vi "DisposeCore.vi"(8 "error in (no error)":errorcluster, 11 "ChicagoStylePepperoniPizza":refnum<class "ChicagoStylePepperoniPizza.lvclass">) -> (0 "error out":errorcluster, 3 "ChicagoStylePepperoniPizza":refnum<class "ChicagoStylePepperoniPizza.lvclass">)   [LabVIEW 2020, in "FactoryMethod.lvlib" / "PizzaFactoryMethod.lvlib" / "ChicagoStylePepperoniPizza.lvclass"]
uses:
  ChicagoStylePepperoniPizza.lvclass
  ChicagoStylePepperoniPizza.lvclass/ChicagoStylePepperoniPizza.ctl
  Private/TypeDef/privateDataDVR.ctl
  Private/TypeDef/privateData.ctl
  Pizza/Pizza.lvclass
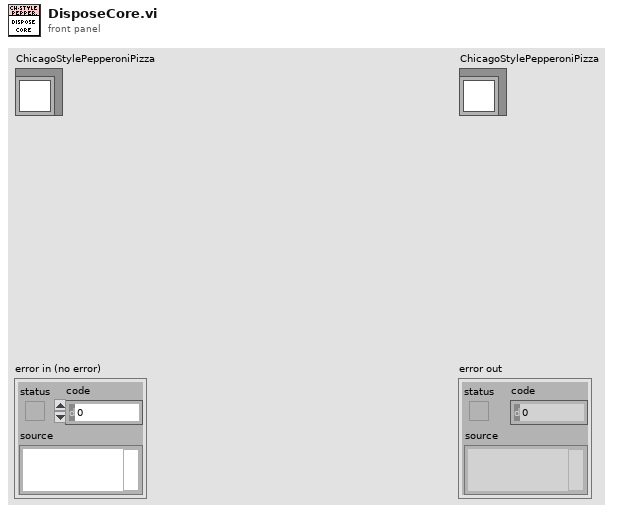
[diagram p1: front panel]
types:
  T1 = typedef "FactoryMethod.lvlib/PizzaFactoryMethod.lvlib/ChicagoStylePepperoniPizza.lvclass/privateDataDVR.ctl" = refnum<data-value>
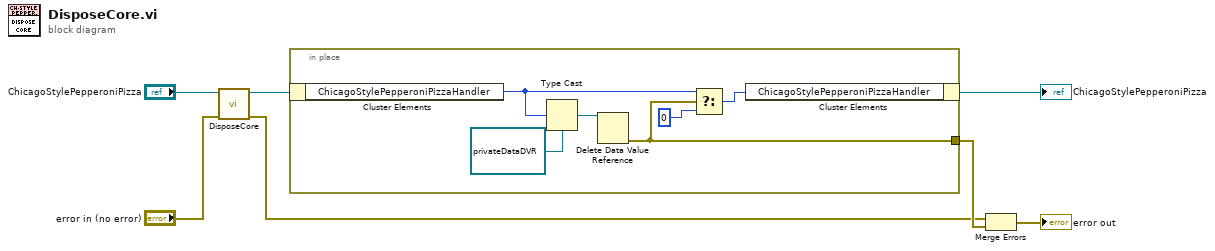
[diagram p0: block diagram]
diagram:
  n1 = call-parent "DisposeCore.vi"("error in"="error in (no error)", "Pizza"="ChicagoStylePepperoniPizza") -> ("error out"=w1:errorcluster, "Pizza"=w3:refnum<class "ChicagoStylePepperoniPizza.lvclass">)  [unwired: 8 in]
  n2 = in-place {
    in-place-border: [w12] -> w5
    n3 = in-place-cluster #1(w3) -> ("ChicagoStylePepperoniPizzaHandler"=w11:u32)
    n4 = Type Cast(type=T1 refnum ("privateDataDVR"), x=w11) -> (*(type *) &x=w13:T1)
    n5 = Delete Data Value Reference(data value reference=w13) -> (error out=w12:errorcluster)  [unwired: 1 in, 1 out]
    n6 = Select(t=w11, s=w12, f=u32 0) -> (s? t:f=w10:u32)
    n7 = in-place-cluster #1("ChicagoStylePepperoniPizzaHandler"=w10) -> (→"ChicagoStylePepperoniPizza":refnum<class "ChicagoStylePepperoniPizza.lvclass">)
  }
  n8 = Merge Errors(w1, w5) -> (→"error out":errorcluster)
